vi "Open HVPS.vi"(8 "error in":errorcluster, 11 "SR 3XX HVPS in":refnum<class "SR 3XX HVPS.lvclass">) -> (0 "error out":errorcluster, 3 "SR 3XX HVPS out":refnum<class "SR 3XX HVPS.lvclass">)   [LabVIEW 2014, in "SR 3XX HVPS.lvclass"]
doc: "Opens a connection to the power supply using the address provided by <B>GPIB Resc</B>."
uses:
  SR 3XX HVPS.lvclass
  SR 3XX HVPS.lvclass/SR 3XX HVPS.ctl
  Read GPIB Addr.vi
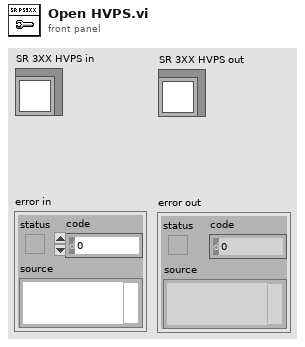
[diagram p1: front panel]
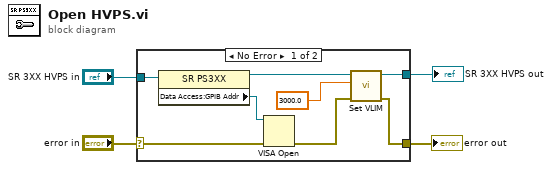
[diagram p0: block diagram]
diagram:
  n1 = case shown="No Error" "error in" {
    selector: "error in" -> [w12 w14]
    tunnel: [w5 w14] -> w3
    tunnel: [w6 w13] -> w1
    tunnel: "SR 3XX HVPS in" -> [w9 w13]
    frame No Error {
      n2 = property class="SR PS3XX"(reference=w9) -> (reference out=w8:refnum<class "SR 3XX HVPS.lvclass">, "Data Access:GPIB Addr"=w7:refnum<visa-resource-name>)  [unwired: 1 in, 1 out]
      n3 = VISA Open(error in (no error)=w12, VISA resource name=w7) -> (error out=w11:errorcluster)  [unwired: 3 in, 1 out]
      n4 = call "Set VLIM.vi"("error in"=w11, "VLIM"=sgl 3000.0, "SR 3XX HVPS in"=w8) -> ("error out"=w5:errorcluster, "SR 3XX HVPS out"=w6:refnum<class "SR 3XX HVPS.lvclass">)  [unwired: 7 in]
    }
    frame Error {
    }
  }
  "error out" <- w3
  "SR 3XX HVPS out" <- w1
